vi "Add.vi"(8 "error in (no error)":errorcluster, 9 "Name":string, 10 "LabVIEW Object":refnum<class>, 11 "CollectionByRef in":refnum<class "CollectionByRef.lvclass">) -> (0 "error out":errorcluster, 3 "CollectionByRef out":refnum<class "CollectionByRef.lvclass">)   [LabVIEW 2021, in "Collection.lvlib" / "CollectionByRef.lvclass"]
uses:
  CollectionByRef.lvclass
  CollectionByRef.lvclass/CollectionByRef.ctl
  CollectionByValue/CollectionByValue.lvclass
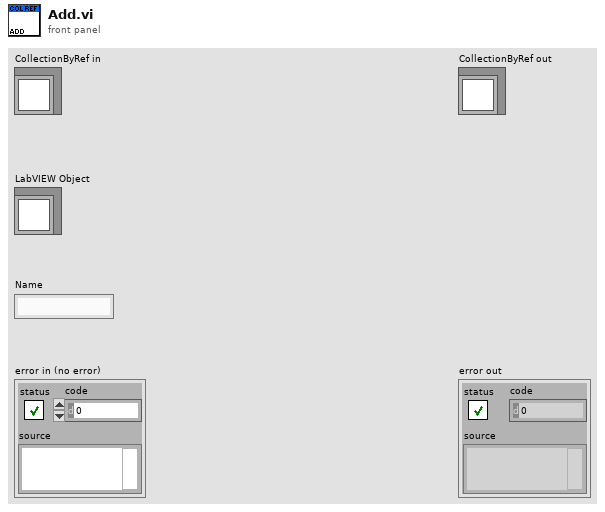
[diagram p1: front panel]
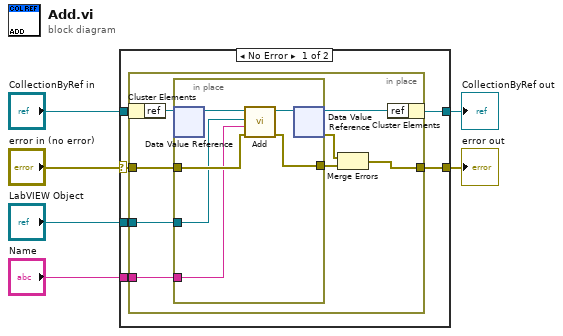
[diagram p0: block diagram]
diagram:
  n1 = case shown="No Error" "error in (no error)" {
    selector: "error in (no error)" -> [w10 w28]
    tunnel: [w9 w28] -> w5
    tunnel: [w11 w27] -> w3
    tunnel: "CollectionByRef in" -> [w12 w27]
    tunnel: "LabVIEW Object" -> [w8 _]
    tunnel: "Name" -> [w7 _]
    frame No Error {
      n2 = in-place {
        in-place-border: w10 -> [w18]
        in-place-border: [w15] -> w9
        in-place-border: w8 -> [w14]
        in-place-border: w7 -> [w13]
        n3 = in-place-cluster #1(w12) -> ("ref"=w19:refnum<data-value>)
        n4 = in-place {
          in-place-border: w18 -> [w24]
          in-place-border: [w23] -> w16
          in-place-border: w14 -> [w22]
          in-place-border: w13 -> [w21]
          n5 = in-place-dvr #2(w19) -> (w26:refnum<class "CollectionByValue.lvclass">)  [unwired: 1 out]
          n6 = call "Add.vi"("error in (no error)"=w24, "Name"=w21, "LabVIEW Object"=w22, "Collection in"=w26) -> ("error out"=w23:errorcluster, "Collection out"=w25:refnum<class "CollectionByValue.lvclass">)  [unwired: 6 in]
          n7 = in-place-dvr #2(w25) -> (w20:refnum<data-value>, w17:errorcluster)
        }
        n8 = Merge Errors(w17, w16) -> (w15:errorcluster)
        n9 = in-place-cluster #1("ref"=w20) -> (w11:refnum<class "CollectionByRef.lvclass">)
      }
    }
    frame Error {
    }
  }
  "error out" <- w5
  "CollectionByRef out" <- w3
